vi "macro_NumCmd_Recv_Generic.vi"() -> ()   [LabVIEW 2019, in "Trajectory_Library.lvlib"]
uses:
  Trajectory_Library.lvlib
  TypeDef/POSE3D.ctl
  TypeDef/TRANSLATION3D.ctl
  TypeDef/ROTATION3D.ctl
  TypeDef/QUATERNION.ctl
  VI/numCmd_ObtainQueue_Generic.vi
panel:
  out "TargetPose":T1={"Translation3d"={"X"=0.0, "Y"=0.0, "Z"=0.0}, "Rotation3d"={"Q_quaternion"={"R"=1.0, "V"=[0.0, 0.0, 0.0]}}} {"Translation3d"."Z" format="%14.3f"; "Translation3d"."Y" format="%14.3f"; "Translation3d"."X" format="%14.3f"}
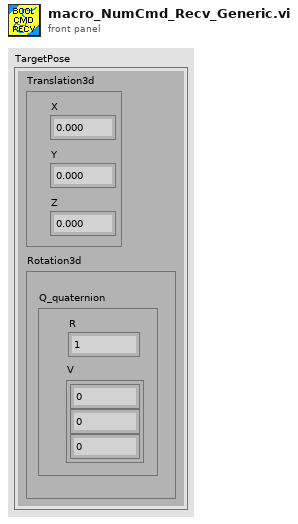
[diagram p1: front panel]
types:
  T1 = typedef "Trajectory_Library.lvlib/POSE3D.ctl" = cluster{"Translation3d":T2, "Rotation3d":T3}
  T2 = typedef "Trajectory_Library.lvlib/TRANSLATION3D.ctl" = cluster{"X":dbl, "Y":dbl, "Z":dbl}
  T3 = typedef "Trajectory_Library.lvlib/ROTATION3D.ctl" = cluster{"Q_quaternion":T4}
  T4 = typedef "Trajectory_Library.lvlib/QUATERNION.ctl" = cluster{"R":dbl, "V":dbl[]}
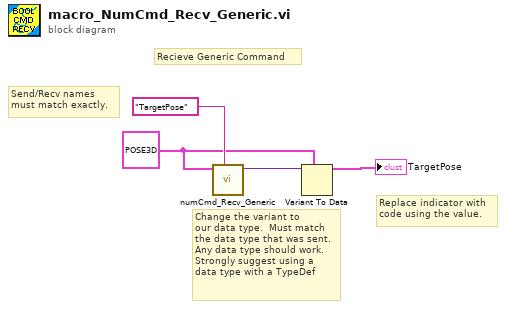
[diagram p0: block diagram]
diagram:
  w1 = T1 {"Translation3d"={"X"=0.0, "Y"=0.0, "Z"=0.0}, "Rotation3d"={"Q_quaternion"={"R"=1.0, "V"=[0.0, 0.0, 0.0]}}} ("POSE3D")
  # "Change the variant to\nour data type.  Must match\nthe data type that was sent.\nAny data type should work.\nStrongly suggest using a \ndata type with a TypeDef"
  # "Send/Recv names\nmust match exactly."
  # "Replace indicator with\ncode using the value."
  # "Recieve Generic Command"
  n1 = call "numCmd_Recv_Generic.vi"("Command Name"="TargetPose", "Initial Value"=w1) -> ("Newest Value"=w3:variant)  [unwired: 7 in, 2 out]
  n2 = Variant To Data(type=w1, Variant=w3) -> (data=→"TargetPose":T1)  [unwired: 1 in, 1 out]
